vi "Close Notifiers.vi"(8 "error in":errorcluster, 11 "Notifiers":T1) -> (0 "error out":errorcluster)   [LabVIEW 2015, in "PLC Notifiers.lvlib"]
uses:
  PLC Notifiers.lvlib
  PLC Notifiers.ctl
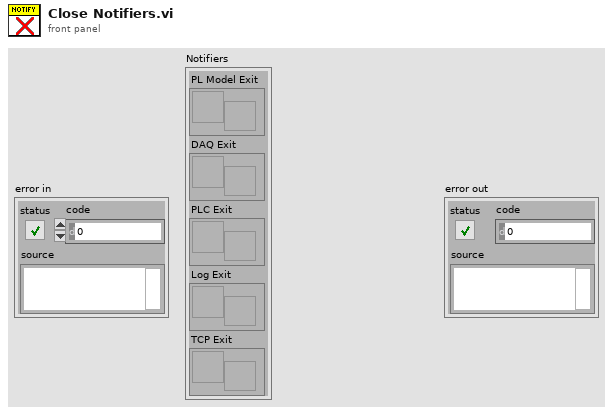
[diagram p1: front panel]
types:
  T1 = typedef "PLC Notifiers.lvlib/PLC Notifiers.ctl" = cluster{"PL Model Exit":refnum<notifier>, "DAQ Exit":refnum<notifier>, "PLC Exit":refnum<notifier>, "Log Exit":refnum<notifier>, "TCP Exit":refnum<notifier>}
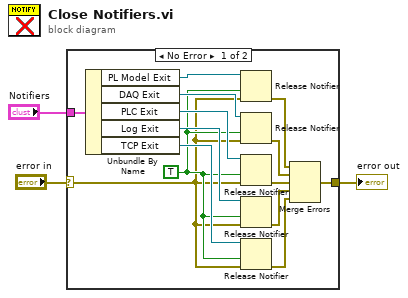
[diagram p0: block diagram]
diagram:
  n1 = case shown="No Error" "error in" {
    selector: "error in" -> [w5 w18]
    tunnel: [w14 w18] -> w2
    tunnel: "Notifiers" -> [w17 _]
    frame No Error {
      w6 = TRUE ("force destroy? (F)")
      n2 = Unbundle By Name(w17) -> ("PL Model Exit"=w16:refnum<notifier>, "DAQ Exit"=w13:refnum<notifier>, "PLC Exit"=w11:refnum<notifier>, "Log Exit"=w8:refnum<notifier>, "TCP Exit"=w7:refnum<notifier>)
      n3 = Release Notifier(notifier=w16, force destroy? (F)=w6, error in (no error)=w5) -> (error out=w15:errorcluster)  [unwired: 2 out]
      n4 = Release Notifier(notifier=w13, force destroy? (F)=w6, error in (no error)=w5) -> (error out=w12:errorcluster)  [unwired: 2 out]
      n5 = Release Notifier(notifier=w11, force destroy? (F)=w6, error in (no error)=w5) -> (error out=w10:errorcluster)  [unwired: 2 out]
      n6 = Release Notifier(notifier=w8, force destroy? (F)=w6, error in (no error)=w5) -> (error out=w9:errorcluster)  [unwired: 2 out]
      n7 = Release Notifier(notifier=w7, force destroy? (F)=w6, error in (no error)=w5) -> (error out=w4:errorcluster)  [unwired: 2 out]
      n8 = Merge Errors(w15, w12, w10, w9, w4) -> (w14:errorcluster)
    }
    frame Error {
    }
  }
  "error out" <- w2
